vi "RGseriesSeria19531Ceramic.vi"() -> ()   [LabVIEW 2015]
uses:
  <vilib>/Instr/_visa.llb/VISA Configure Serial Port (Instr).vi
  <userlib>/caLab/Private/Get_PV-1D.vi
  <userlib>/caLab/Private/Get_PV.vi
  <userlib>/caLab/Private/Put_DBL-1D_PV-1D.vi
panel:
  in  "Ifactor":dbl=33.3
  in  "APX:PS2_T_RV":dbl
  out "APX:PS2_V_EV":dbl format="%.3f"
  out "APX:PS2_I_EV":dbl format="%.3f"
  out "Ilim_factor":dbl
  out "Vlim_factor":dbl
  out "SSE:Tsample":dbl
  in  "I lower limit":dbl
  in  "V lower limit":dbl
  in  "I upper limit":dbl=2.8
  in  "V upper limit":dbl=18.0
  out "APX:PS2_Ct":dbl
  out "APX:PS2_Rzero":dbl
  in  "Heater":u16(ring) items=["Ceramic W/Mo", "Kanthal A-1"]
  out "APX:Theater":dbl
  out "APX:PS2_R_MV":dbl format="%.2f"
  out "PS1:R_MV":dbl format="%.2f"
  out "APX:Tpiezo":dbl
  in  "REMOTE/LOCAL":bool
  out "APX:Tcopper":dbl
  in  "Timer1":bool
  in  "Reset Timer1":bool=TRUE caption="Auto Reset"
  out "Time has Elapsed":bool
  in  "Time Target1 (min)":dbl=1.0 caption="Time Target (s)"
  out "Elapsed Time (min)":dbl caption="Elapsed Time (s)"
  in  "PS1:I_RV":dbl min=0.0 max=0.5 step=0.01
  in  "PS1:V_RV":dbl min=0.0 max=5.0 step=0.01
  out "PS1:P_MV":dbl format="%.2f"
  out "PS1:I_MV":dbl format="%.3g"
  out "PS1:V_MV":dbl format="%.3g"
  in  "PS1:OUT":bool
  out "APX:Thpc OK?":bool
  out "APX:Tpiezo OK?":bool
  out "PS2_P_MV":dbl format="%.2f"
  in  "APX:PS2_I_RV":dbl min=0.0 max=0.5 step=0.002
  in  "APX:PS2_OUT":bool
  in  "stop":bool
  out "APX:PS2_I_MV":dbl format="%.3g"
  out "APX:PS2_V_MV":dbl format="%.3g"
  in  "VISA resource name":refnum<visa-resource-name>="COM12"
  in  "APX:PS2_V_RV":dbl min=0.0 max=8.0 step=0.05
  # "Sample Heater Control"
  # "Copper mesh temperature control"
  # "COM12"
  # "V"
  # "V"
  # "A"
  # "A"
  # "Max 1.2A/0.4x0.1wire"
  # "W"
  # "ohm"
  # "W"
  # "ohm"
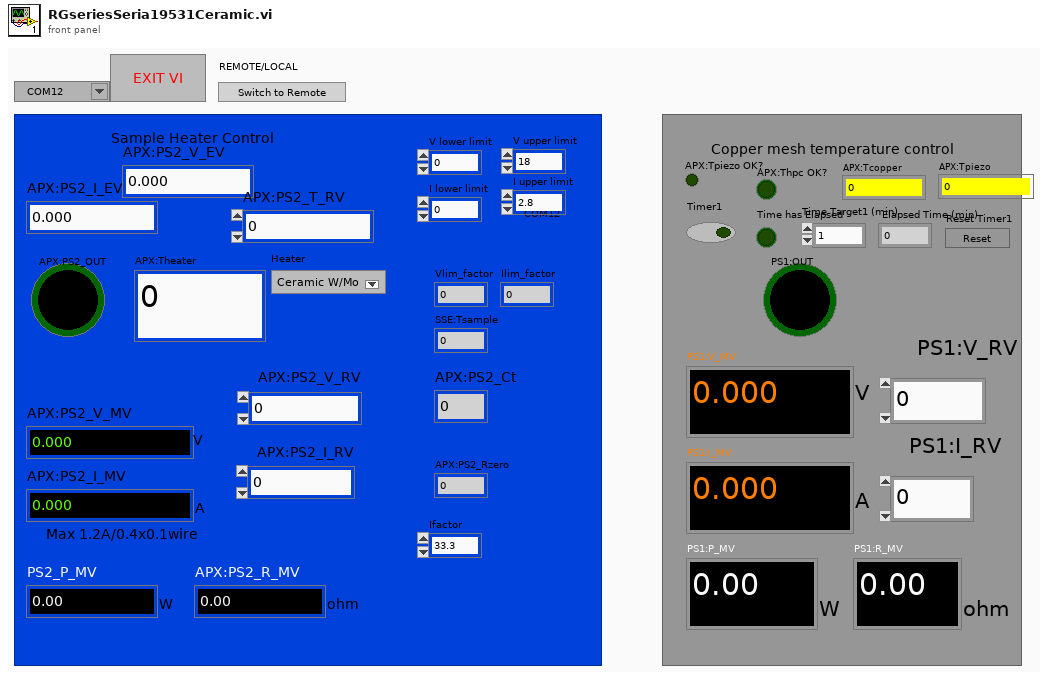
[diagram p1: front panel]
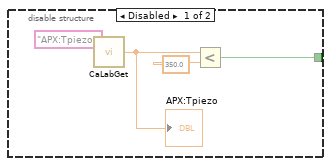
[diagram p2: hidden frame]
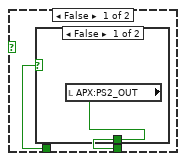
[diagram p4: hidden frame]
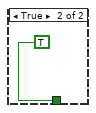
[diagram p5: hidden frame]
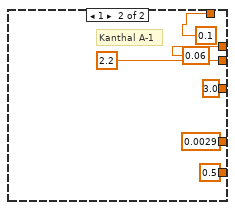
[diagram p6: hidden frame]
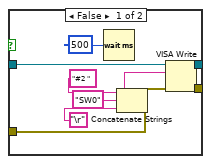
[diagram p7: hidden frame]
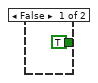
[diagram p9: hidden frame]
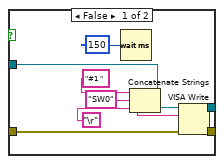
[diagram p10: hidden frame]
diagram:
  w45 = u16 0 items=["None", "XON/XOFF", "RTS/CTS", "XON/XOFF & RTS/CTS", "DTR/DSR", "XON/XOFF & DTR/DSR"] ("flow control (0:none)")
  w46 = u16 10 items=["1.0"=10, "1.5"=15, "2.0"=20] ("stop bits (10: 1 bit)")
  # "enable output"
  # "disable remote control"
  # "OpenComport"
  # "Stop bits"
  # "enable remote control"
  # "enable output"
  n1 = Concatenate Strings("#2 " ("initial string"), "REN" ("string"), "\r") -> (w44:string)
  n2 = call-poly "VISA Configure Serial Port"("VISA resource name"="VISA resource name", "timeout (10sec)"=u32 10000, "baud rate (9600)"=u32 9600, "data bits (8)"=u16 8, "parity (0:none)"=enum16{"None", "Odd", "Even", "Mark", "Space"}."None", "stop bits (10: 1 bit)"=w46, "flow control (0:none)"=w45) -> ("VISA resource name out"=w41:refnum<visa-resource-name>, "error out"=w40:errorcluster)  [unwired: 7 in]
  n3 = VISA Write(VISA resource name=w41, write buffer=w44, error in (no error)=w40) -> (VISA resource name out=w10:refnum<visa-resource-name>, error out=w3:errorcluster)  [unwired: 1 out]
  n4 = flat-sequence {
    tunnel: w3 -> [w60]
    tunnel: [w60] -> w4
    frame #0 {
      n5 = Wait (ms)(milliseconds to wait=u32 500) -> ()  [unwired: 1 out]
    }
  }
  n6 = Concatenate Strings("#1 " ("initial string"), "REN" ("string"), "\r") -> (w5:string)
  n7 = VISA Write(VISA resource name=w10, write buffer=w5, error in (no error)=w4) -> (VISA resource name out=w9:refnum<visa-resource-name>, error out=w2:errorcluster)  [unwired: 1 out]
  n8 = flat-sequence {
    tunnel: [w64] -> w27
    tunnel: w2 -> [w64]
    frame #0 {
      n9 = Wait (ms)(milliseconds to wait=u32 500) -> ()  [unwired: 1 out]
      n10 = property on="APX:PS2_V_RV" class="DigNum (strict)"("Value"=0.0 ("VCN_REQ")) -> ()  [unwired: 2 in, 2 out]
      n11 = property on="APX:PS2_I_RV" class="DigNum (strict)"("Value"=0.0 ("APX:RG183_I_RV")) -> ()  [unwired: 2 in, 2 out]
    }
  }
  n12 = local write "REMOTE/LOCAL"(FALSE ("REMOTE/LOCAL")) -> ()
  n13 = Concatenate Strings("#2 " ("format string"), "SW0" ("initial string"), "\r" ("input 1")) -> (w43:string)
  n14 = VISA Write(VISA resource name=w9, write buffer=w43, error in (no error)=w27) -> (VISA resource name out=w29:refnum<visa-resource-name>, error out=w28:errorcluster)  [unwired: 1 out]
  n15 = while {
    tunnel: w29 -> [w74]
    tunnel: w28 -> [w75]
    tunnel: [w71] -> w26
    tunnel: [w70] -> w25
    stop <- "stop" stop-if-true
    n16 = flat-sequence {
      tunnel: w74 -> [w85]
      tunnel: w75 -> [w86]
      tunnel: [w86] -> w68
      tunnel: [w85] -> w67
      tunnel: [w167] -> w73
      tunnel: [w166] -> w72
      tunnel: w68 -> [w165]
      tunnel: w67 -> [w163]
      tunnel: w73 -> [w300]
      tunnel: w72 -> [w297]
      tunnel: [w278] -> w66
      tunnel: [w277] -> w65
      tunnel: [w394] -> w70
      tunnel: [w395] -> w71
      tunnel: w66 -> [w395]
      tunnel: w65 -> [w394]
      frame #0 {
        n17 = disable-structure shown="Enabled" {
          disable-tunnel: [w87 TRUE ("APX:Tpiezo OK?")] -> w78
          frame Disabled {
            n18 = call-poly <userlib>:"CaLabGet.vi"("PV Name"="APX:Tpiezo") -> ("1rst Value (number)"=w89:dbl)  [unwired: 8 in, 6 out]
            "APX:Tpiezo" <- w89
            n19 = Less?(x=w89, y=350.0) -> (x < y?=w87:bool)
          }
          frame Enabled {
          }
        }
        "APX:Tpiezo OK?" <- w78
        n20 = case shown="0, Default" "Heater" {
          tunnel: [0.00483 ("APX:PS2_Ct") 0.0029 ("APX:PS2_Ct")] -> w81
          tunnel: [9.3 ("APX:PS2_Rzero") 0.5 ("APX:PS2_Rzero")] -> w82
          tunnel: [0.5 2.2] -> w83
          tunnel: [10.0 3.0] -> w84
          tunnel: [0.1 0.1] -> w77
          tunnel: [0.06 0.06] -> w76
          frame 0, Default {
            (unwired) 9.89 ("APX:PS2_Rzero")
            (unwired) 0.0325 ("APX:PS2_Ct")
            (unwired) 6.21 ("APX:PS2_Rzero")
            # "W/Mo"
          }
          frame 1 {
            # "Kanthal A-1"
          }
        }
        n21 = case shown="True" "REMOTE/LOCAL" {
          frame False {
          }
          frame True {
            w94 = 0 ("disabled index (col)")
            (unwired) "APX:Thpc"
            n22 = call-poly <userlib>:"CaLabGet.vi"("PV Names"=string[] ["APX:PS2_V_RV", "APX:PS2_I_RV", "APX:PS2_OUT_1", "APX:PS2_OUT_0", "SSE:Tsample"]) -> ("Value Array (number)"=w93:dbl[][])  [unwired: 8 in, 6 out]
            n23 = Index Array(array=w93, index (row)=4, index (col)=w94) -> (element=→"SSE:Tsample":dbl)
            n24 = Index Array(array=w93, index (row)=2, index (col)=w94) -> (element=w107:dbl)
            n25 = Index Array(array=w93, index (row)=0, index (col)=w94) -> (element=w97:dbl)
            n26 = Index Array(array=w93, index (row)=1, index (col)=w94) -> (element=w96:dbl)
            n27 = Index Array(array=w93, index (row)=3 ("disabled index (row)"), index (col)=w94) -> (element=w101:dbl)
            n28 = Number To Boolean Array(number=w107) -> (Boolean array=w106:bool[])
            n29 = Number To Boolean Array(number=w101) -> (Boolean array=w103:bool[])
            n30 = local write "APX:PS2_I_RV"(w96) -> ()
            n31 = Index Array(array=w106, index=0) -> (element=w99:bool)
            n32 = local write "APX:PS2_V_RV"(w97) -> ()
            n33 = Index Array(array=w103, index=0) -> (element=w100:bool)
            n34 = case shown="True" w100 {
              tunnel: w99 -> [w113 _]
              tunnel: [w112 FALSE] -> w98
              frame False {
                n35 = case shown="False" w113 {
                  tunnel: [w114 TRUE] -> w112
                  frame False {
                    n36 = local read "APX:PS2_OUT"() -> (w114:bool)
                  }
                  frame True {
                  }
                }
              }
              frame True {
              }
            }
            n37 = local write "APX:PS2_OUT"(w98) -> ()
          }
        }
        n38 = local write "I upper limit"(w83) -> ()
        n39 = local write "V upper limit"(w84) -> ()
        n40 = local write "APX:PS2_Ct"(w81) -> ()
        n41 = local write "APX:PS2_Rzero"(w82) -> ()
        n42 = local write "V lower limit"(w77) -> ()
        n43 = local write "I lower limit"(w76) -> ()
      }
      frame #1 {
        w139 = 293.0 ("y")
        # "measure current"
        # "measure voltage"
        # "measure voltage"
        # "measure curent"
        # "Measured Voltage"
        # "Measured Current"
        # "Set current"
        # "Set voltage"
        # "disable output"
        n44 = local read "APX:PS2_Rzero"() -> (w134:dbl)
        n45 = local read "APX:PS2_R_MV"() -> (w152:dbl)
        n46 = In Range and Coerce(upper limit=65.0, x=w152, lower limit=w134) -> (coerced(x)=w150:dbl)  [unwired: 1 out]
        n47 = Divide(x=w150, y=w134) -> (x/y=w149:dbl)
        n48 = Subtract(x="APX:PS2_T_RV", y=w139) -> (x-y=w133:dbl)
        n49 = Subtract(x=w149, y=1.0) -> (x-y=w147:dbl)
        n50 = local read "APX:PS2_Ct"() -> (w138:dbl)
        n51 = Multiply(x=w133, y=w138) -> (x*y=w137:dbl)
        n52 = Divide(x=w147, y=w138) -> (x/y=w146:dbl)
        n53 = Add(x=w137, y=1.0) -> (x+y=w135:dbl)
        n54 = Multiply(x=w135, y=w134) -> (x*y=w130:dbl)
        n55 = Multiply(x=w133, y=0.02) -> (x*y=w129:dbl)
        "APX:PS2_V_EV" <- w129
        n56 = Add(x=w146, y=w139) -> (x+y=→"APX:Theater":dbl)
        n57 = Divide(x=w129, y=w130) -> (x/y=→"APX:PS2_I_EV":dbl)
        n58 = case shown="True" "APX:PS2_OUT" {
          tunnel: w163 -> [w233 w242]
          tunnel: w165 -> [w232 w241]
          tunnel: [w231 w240] -> w164
          tunnel: [w230 w239] -> w162
          frame False {
            n59 = Wait (ms)(milliseconds to wait=u32 500) -> ()  [unwired: 1 out]
            n60 = Concatenate Strings("#2 " ("format string"), "SW0" ("initial string"), "\r" ("input 1")) -> (w235:string)
            n61 = VISA Write(VISA resource name=w233, write buffer=w235, error in (no error)=w232) -> (VISA resource name out=w230:refnum<visa-resource-name>, error out=w231:errorcluster)  [unwired: 1 out]
          }
          frame True {
            n62 = Wait (ms)(milliseconds to wait=u32 150) -> ()  [unwired: 1 out]
            n63 = Concatenate Strings("#2 " ("format string"), "SW1" ("initial string"), "\r" ("input 1")) -> (w244:string)
            n64 = VISA Write(VISA resource name=w242, write buffer=w244, error in (no error)=w241) -> (VISA resource name out=w239:refnum<visa-resource-name>, error out=w240:errorcluster)  [unwired: 1 out]
          }
        }
        n65 = In Range and Coerce(upper limit="V upper limit", x="APX:PS2_V_RV", lower limit="V lower limit") -> (coerced(x)=w160:dbl)  [unwired: 1 out]
        n66 = flat-sequence {
          tunnel: w162 -> [w260]
          tunnel: w164 -> [w261]
          tunnel: [w261] -> w168
          tunnel: [w260] -> w169
          frame #0 {
            n67 = Wait (ms)(milliseconds to wait=u32 150) -> ()  [unwired: 1 out]
          }
        }
        n68 = Multiply(x=5.5, y=w160) -> (x*y=w227:dbl)
        n69 = Number To Fractional String(number=w227, width (-)=i16 5, precision (6)=i16 2) -> (F-format string=w228:string)  [unwired: 1 in]
        n70 = Concatenate Strings("#2" ("format string"), "VCN " ("initial string"), w228, "\r") -> (w173:string)
        n71 = Concatenate Strings("#2 " ("format string"), "VM" ("initial string"), "\r" ("input 1")) -> (w204:string)
        n72 = VISA Write(VISA resource name=w169, write buffer=w173, error in (no error)=w168) -> (VISA resource name out=w203:refnum<visa-resource-name>, error out=w202:errorcluster)  [unwired: 1 out]
        n73 = VISA Write(VISA resource name=w203, write buffer=w204, error in (no error)=w202) -> (VISA resource name out=w189:refnum<visa-resource-name>, error out=w187:errorcluster)  [unwired: 1 out]
        n74 = flat-sequence {
          tunnel: w189 -> [w259]
          tunnel: [w259] -> w188
          tunnel: w187 -> [w258]
          tunnel: [w258] -> w186
          frame #0 {
            n75 = Wait (ms)(milliseconds to wait=u32 150) -> ()  [unwired: 1 out]
          }
        }
        n76 = In Range and Coerce(upper limit="I upper limit", x="APX:PS2_I_RV", lower limit="I lower limit") -> (coerced(x)=w158:dbl)  [unwired: 1 out]
        n77 = Multiply(x=33.0, y=w158) -> (x*y=w217:dbl)
        n78 = property class="Instr"(reference=w188, error in=w186) -> (reference out=w195:refnum<visa-resource-name>, error out=w194:errorcluster, "Serial Settings:Number of Bytes at Serial Port"=w193:u32)
        n79 = Number To Fractional String(number=w217, width (-)=i16 5, precision (6)=i16 2) -> (F-format string=w220:string)  [unwired: 1 in]
        n80 = VISA Read(VISA resource name=w195, byte count=w193, error in (no error)=w194) -> (VISA resource name out=w181:refnum<visa-resource-name>, read buffer=w174:string, error out=w180:errorcluster)  [unwired: 1 out]
        n81 = flat-sequence {
          tunnel: w181 -> [w252]
          tunnel: w180 -> [w251]
          tunnel: [w252] -> w178
          tunnel: [w251] -> w179
          frame #0 {
            n82 = Wait (ms)(milliseconds to wait=u32 150) -> ()  [unwired: 1 out]
          }
        }
        n83 = Concatenate Strings("#2 " ("initial string"), "ICN " ("initial string"), w220, "\r") -> (w172:string)
        n84 = String Subset(string=w174, offset (0)=3) -> (substring=w171:string)  [unwired: 1 in]
        n85 = Concatenate Strings("#2 " ("format string"), "IM" ("initial string"), "\r" ("input 1")) -> (w197:string)
        n86 = VISA Write(VISA resource name=w178, write buffer=w172, error in (no error)=w179) -> (VISA resource name out=w199:refnum<visa-resource-name>, error out=w200:errorcluster)  [unwired: 1 out]
        n87 = Fract/Exp String To Number(string=w171) -> (number=w213:dbl)  [unwired: 3 in, 1 out]
        n88 = VISA Write(VISA resource name=w199, write buffer=w197, error in (no error)=w200) -> (VISA resource name out=w185:refnum<visa-resource-name>, error out=w184:errorcluster)  [unwired: 1 out]
        n89 = Divide(x=w213, y=5.5 ("x")) -> (x/y=w155:dbl)
        "APX:PS2_V_MV" <- w155
        n90 = flat-sequence {
          tunnel: w185 -> [w255]
          tunnel: w184 -> [w254]
          tunnel: [w255] -> w183
          tunnel: [w254] -> w182
          frame #0 {
            n91 = Wait (ms)(milliseconds to wait=u32 150) -> ()  [unwired: 1 out]
          }
        }
        n92 = property class="Instr"(reference=w183, error in=w182) -> (reference out=w192:refnum<visa-resource-name>, error out=w191:errorcluster, "Serial Settings:Number of Bytes at Serial Port"=w190:u32)
        n93 = VISA Read(VISA resource name=w192, byte count=w190, error in (no error)=w191) -> (VISA resource name out=w177:refnum<visa-resource-name>, read buffer=w175:string, error out=w176:errorcluster)  [unwired: 1 out]
        n94 = flat-sequence {
          tunnel: w177 -> [w249]
          tunnel: w176 -> [w248]
          tunnel: [w249] -> w167
          tunnel: [w248] -> w166
          frame #0 {
            n95 = Wait (ms)(milliseconds to wait=u32 150) -> ()  [unwired: 1 out]
          }
        }
        n96 = String Subset(string=w175, offset (0)=3) -> (substring=w170:string)  [unwired: 1 in]
        n97 = Fract/Exp String To Number(string=w170) -> (number=w210:dbl)  [unwired: 3 in, 1 out]
        n98 = Divide(x=w210, y=33.5 ("x")) -> (x/y=w156:dbl)
        "APX:PS2_I_MV" <- w156
        n99 = Multiply(x=w155, y=w156) -> (x*y=→"PS2_P_MV":dbl)
        n100 = Divide(x=w155, y=w156) -> (x/y=→"APX:PS2_R_MV":dbl)
      }
      frame #2 {
        (unwired) 33.3 ("x")
        (unwired) 37.35 ("x")
        # "measure curent"
        # "Measured Voltage"
        # "Measured Current"
        # "disable output"
        # "measure current"
        # "measure voltage"
        # "Set current"
        # "measure voltage"
        # "Set voltage"
        n101 = case shown="True" "Reset Timer1" {
          frame False {
          }
          frame True {
            n102 = property on="Elapsed Time (min)" class="DigNum (strict)"("Value"=0.0 ("Elapsed Time (min)")) -> ()  [unwired: 2 in, 2 out]
          }
        }
        n103 = case shown="True" "Timer1" {
          tunnel: "Time Target1 (min)" -> [_ w355]
          tunnel: [TRUE w354] -> w268
          frame False {
          }
          frame True {
            w359 = 60.0 ("y")
            n104 = Multiply(x=w355, y=w359) -> (x*y=w357:dbl)
            n105 = call "Elapsed Time"("Time Target (s)"=w357) -> ("Elapsed Time (s)"=w358:dbl, "Time has Elapsed"=w356:bool)  [unwired: 11 in, 6 out]
            "Time has Elapsed" <- w356
            n106 = Divide(x=w358, y=w359) -> (x/y=→"Elapsed Time (min)":dbl)
            n107 = Not(x=w356) -> (.not. x?=w354:bool)
          }
        }
        n108 = call-poly <userlib>:"CaLabGet.vi"("PV Name"="APX:Tcopper") -> ("1rst Value (number)"=w350:dbl)  [unwired: 8 in, 6 out]
        "APX:Tcopper" <- w350
        n109 = Less?(x=w350, y=420.0) -> (x < y?=w299:bool)
        "APX:Thpc OK?" <- w299
        n110 = And(x=w299, y="PS1:OUT") -> (x .and. y?=w272:bool)
        n111 = And(x=w272, y=w268) -> (x .and. y?=w271:bool)
        n112 = case shown="True" w271 {
          tunnel: w300 -> [w373 w382]
          tunnel: w297 -> [w372 w381]
          tunnel: [w371 w380] -> w296
          tunnel: [w370 w379] -> w295
          frame False {
            n113 = Wait (ms)(milliseconds to wait=u32 150) -> ()  [unwired: 1 out]
            n114 = Concatenate Strings("#1 " ("format string"), "SW0" ("initial string"), "\r" ("input 1")) -> (w377:string)
            n115 = VISA Write(VISA resource name=w373, write buffer=w377, error in (no error)=w372) -> (VISA resource name out=w370:refnum<visa-resource-name>, error out=w371:errorcluster)  [unwired: 1 out]
          }
          frame True {
            n116 = Wait (ms)(milliseconds to wait=u32 150) -> ()  [unwired: 1 out]
            n117 = Concatenate Strings("#1 " ("format string"), "SW1" ("initial string"), "\r" ("input 1")) -> (w386:string)
            n118 = VISA Write(VISA resource name=w382, write buffer=w386, error in (no error)=w381) -> (VISA resource name out=w379:refnum<visa-resource-name>, error out=w380:errorcluster)  [unwired: 1 out]
          }
        }
        n119 = In Range and Coerce(upper limit=5.01, x="PS1:V_RV", lower limit=0.0) -> (coerced(x)=w312:dbl)  [unwired: 1 out]
        n120 = flat-sequence {
          tunnel: [w389] -> w293
          tunnel: w296 -> [w389]
          tunnel: [w388] -> w294
          tunnel: w295 -> [w388]
          frame #0 {
            n121 = Wait (ms)(milliseconds to wait=u32 150) -> ()  [unwired: 1 out]
          }
        }
        n122 = Multiply(x=5.55, y=w312) -> (x*y=w303:dbl)
        n123 = Number To Fractional String(number=w303, width (-)=i16 5, precision (6)=i16 2) -> (F-format string=w302:string)  [unwired: 1 in]
        n124 = Concatenate Strings("#1" ("format string"), "VCN " ("initial string"), w302, "\r") -> (w317:string)
        n125 = Concatenate Strings("#1" ("format string"), "VM" ("initial string"), "\r" ("input 1")) -> (w316:string)
        n126 = VISA Write(VISA resource name=w294, write buffer=w317, error in (no error)=w293) -> (VISA resource name out=w318:refnum<visa-resource-name>, error out=w344:errorcluster)  [unwired: 1 out]
        n127 = VISA Write(VISA resource name=w318, write buffer=w316, error in (no error)=w344) -> (VISA resource name out=w345:refnum<visa-resource-name>, error out=w346:errorcluster)  [unwired: 1 out]
        n128 = flat-sequence {
          tunnel: w345 -> [w393]
          tunnel: [w393] -> w347
          tunnel: w346 -> [w392]
          tunnel: [w392] -> w348
          frame #0 {
            n129 = Wait (ms)(milliseconds to wait=u32 150) -> ()  [unwired: 1 out]
          }
        }
        n130 = property class="Instr"(reference=w347, error in=w348) -> (reference out=w340:refnum<visa-resource-name>, error out=w341:errorcluster, "Serial Settings:Number of Bytes at Serial Port"=w342:u32)
        n131 = VISA Read(VISA resource name=w340, byte count=w342, error in (no error)=w341) -> (VISA resource name out=w276:refnum<visa-resource-name>, read buffer=w343:string, error out=w274:errorcluster)  [unwired: 1 out]
        n132 = flat-sequence {
          tunnel: w276 -> [w363]
          tunnel: [w363] -> w275
          tunnel: [w361] -> w273
          tunnel: w274 -> [w361]
          frame #0 {
            n133 = Wait (ms)(milliseconds to wait=u32 150) -> ()  [unwired: 1 out]
          }
        }
        n134 = String Subset(string=w343, offset (0)=3) -> (substring=w332:string)  [unwired: 1 in]
        n135 = In Range and Coerce(upper limit=0.501, x="PS1:I_RV", lower limit=0.0) -> (coerced(x)=w336:dbl)  [unwired: 1 out]
        n136 = Fract/Exp String To Number(string=w332) -> (number=w326:dbl)  [unwired: 3 in, 1 out]
        n137 = Multiply(x="Ifactor", y=w336) -> (x*y=w322:dbl)
        n138 = Number To Fractional String(number=w322, width (-)=i16 5, precision (6)=i16 2) -> (F-format string=w320:string)  [unwired: 1 in]
        n139 = Concatenate Strings("#1 " ("initial string"), "ICN " ("initial string"), w320, "\r") -> (w337:string)
        n140 = Concatenate Strings("#1 " ("format string"), "IM" ("initial string"), "\r" ("input 1")) -> (w338:string)
        n141 = VISA Write(VISA resource name=w275, write buffer=w337, error in (no error)=w273) -> (VISA resource name out=w339:refnum<visa-resource-name>)  [unwired: 2 out]
        n142 = VISA Write(VISA resource name=w339, write buffer=w338) -> (VISA resource name out=w281:refnum<visa-resource-name>, error out=w280:errorcluster)  [unwired: 1 in, 1 out]
        n143 = flat-sequence {
          tunnel: w281 -> [w368]
          tunnel: w280 -> [w367]
          tunnel: [w368] -> w287
          tunnel: [w367] -> w286
          frame #0 {
            n144 = Wait (ms)(milliseconds to wait=u32 150) -> ()  [unwired: 1 out]
          }
        }
        n145 = property class="Instr"(reference=w287, error in=w286) -> (reference out=w290:refnum<visa-resource-name>, error out=w289:errorcluster, "Serial Settings:Number of Bytes at Serial Port"=w288:u32)
        n146 = VISA Read(VISA resource name=w290, byte count=w288, error in (no error)=w289) -> (VISA resource name out=w285:refnum<visa-resource-name>, read buffer=w283:string, error out=w284:errorcluster)  [unwired: 1 out]
        n147 = flat-sequence {
          tunnel: w285 -> [w365]
          tunnel: w284 -> [w364]
          tunnel: [w365] -> w278
          tunnel: [w364] -> w277
          frame #0 {
            n148 = Wait (ms)(milliseconds to wait=u32 150) -> ()  [unwired: 1 out]
          }
        }
        n149 = String Subset(string=w283, offset (0)=3) -> (substring=w282:string)  [unwired: 1 in]
        n150 = Fract/Exp String To Number(string=w282) -> (number=w292:dbl)  [unwired: 3 in, 1 out]
        n151 = Divide(x=w326, y=5.55 ("x")) -> (x/y=w266:dbl)
        "PS1:V_MV" <- w266
        n152 = Divide(x=w292, y="Ifactor") -> (x/y=w265:dbl)
        "PS1:I_MV" <- w265
        n153 = Divide(x=w266, y=w265) -> (x/y=→"PS1:R_MV":dbl)
        n154 = Multiply(x=w266, y=w265) -> (x*y=→"PS1:P_MV":dbl)
      }
      frame #3 {
        n155 = flat-sequence {
          frame #0 {
            w400 = 0.0 ("element")
            n156 = local read "APX:PS2_OUT"() -> (w404:bool)
            n157 = local read "APX:PS2_R_MV"() -> (w409:dbl)
            n158 = local read "APX:PS2_V_MV"() -> (w407:dbl)
            n159 = local read "APX:PS2_I_MV"() -> (w408:dbl)
            n160 = local read "APX:Theater"() -> (w410:dbl)
            n161 = Boolean To (0,1)(Boolean=w404) -> (0, 1=w403:i16)
            n162 = local read "APX:PS2_Rzero"() -> (w396:dbl)
            n163 = Build Array("APX:Theater", "APX:PS2_R_MV", "APX:PS2_I_MV", "APX:PS2_V_MV", "APX:PS2_OUT", "APX:PS2_OUT_0", "APX:PS2_OUT_1", "APX:PS2_Rzero", "APX:PS2_Ct") -> (w415:string[])
            n164 = local read "APX:PS2_Ct"() -> (w397:dbl)
            n165 = Build Array(w410, w409, w408, w407, w403, w400, w400, w396, w397) -> (w406:dbl[])
            n166 = call-poly "CaLabPut.vi"("Values"=w406, "PV Names"=w415) -> ()  [unwired: 6 in, 4 out]
          }
        }
      }
    }
  }
  n167 = Concatenate Strings("#2 " ("format string"), "SW0" ("initial string"), "\r" ("input 1")) -> (w35:string)
  n168 = VISA Write(VISA resource name=w26, write buffer=w35, error in (no error)=w25) -> (VISA resource name out=w31:refnum<visa-resource-name>, error out=w30:errorcluster)  [unwired: 1 out]
  n169 = Concatenate Strings("#2 " ("initial string"), "\r", "GTL" ("input 1")) -> (w42:string)
  n170 = VISA Write(VISA resource name=w31, write buffer=w42, error in (no error)=w30) -> (VISA resource name out=w14:refnum<visa-resource-name>, error out=w13:errorcluster)  [unwired: 1 out]
  n171 = Concatenate Strings("#1 " ("format string"), "SW0" ("initial string"), "\r" ("input 1")) -> (w20:string)
  n172 = VISA Write(VISA resource name=w14, write buffer=w20, error in (no error)=w13) -> (VISA resource name out=w16:refnum<visa-resource-name>, error out=w15:errorcluster)  [unwired: 1 out]
  n173 = Concatenate Strings("#1" ("initial string"), "\r", "GTL" ("input 1")) -> (w21:string)
  n174 = VISA Write(VISA resource name=w16, write buffer=w21, error in (no error)=w15) -> (VISA resource name out=w12:refnum<visa-resource-name>, error out=w11:errorcluster)  [unwired: 1 out]
  n175 = flat-sequence {
    tunnel: w12 -> [w420]
    tunnel: w11 -> [w419]
    tunnel: [w420] -> w37
    tunnel: [w419] -> w36
    frame #0 {
      n176 = Wait (ms)(milliseconds to wait=u32 100) -> ()  [unwired: 1 out]
      n177 = property on="APX:PS2_OUT" class="Bool (strict)"("Value"=FALSE ("Output")) -> ()  [unwired: 2 in, 2 out]
      n178 = property on="APX:PS2_V_RV" class="DigNum (strict)"("Value"=0.0 ("VCN_REQ")) -> ()  [unwired: 2 in, 2 out]
      n179 = property on="APX:PS2_I_RV" class="DigNum (strict)"("Value"=0.0 ("APX:RG183_I_RV")) -> ()  [unwired: 2 in, 2 out]
    }
  }
  n180 = VISA Close(VISA resource name=w37, error in (no error)=w36) -> ()  [unwired: 1 out]
